vi "Write Balance.vi"(8 "error in (no error)":errorcluster, 10 "Balance":dbl, 11 "AAccount in":refnum<class "AAccount.lvclass">) -> (0 "error out":errorcluster, 3 "AAccount out":refnum<class "AAccount.lvclass">)   [LabVIEW 2020, in "AAccount.lvclass"]
uses:
  AAccount.lvclass
  AAccount.lvclass/AAccount.ctl
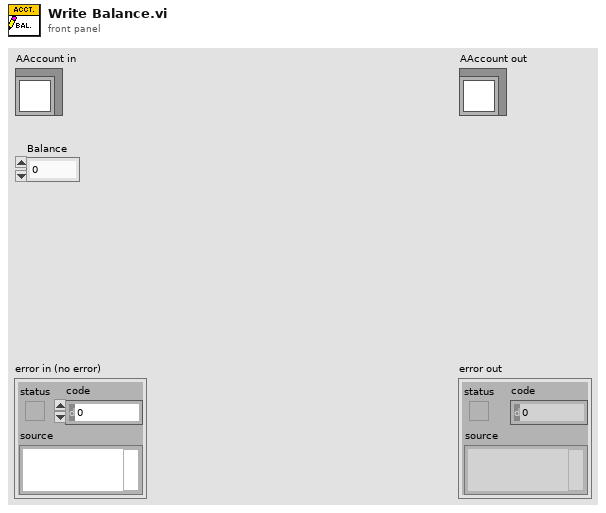
[diagram p1: front panel]
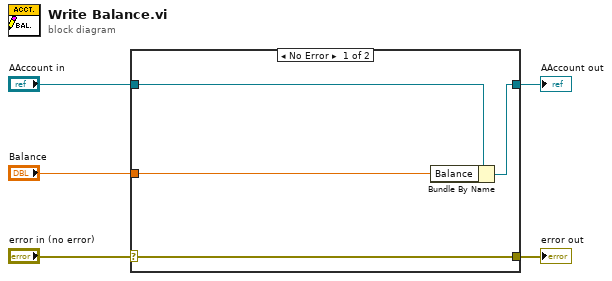
[diagram p0: block diagram]
diagram:
  n1 = case shown="No Error" "error in (no error)" {
    selector: "error in (no error)" -> [w9 w10]
    tunnel: [w9 w10] -> w4
    tunnel: [w7 w11] -> w2
    tunnel: "AAccount in" -> [w8 w11]
    tunnel: "Balance" -> [w6 _]
    frame No Error {
      n2 = Bundle By Name(cluster=w8, "Balance"=w6) -> (w7:refnum<class "AAccount.lvclass">)
    }
    frame Error {
    }
  }
  "error out" <- w4
  "AAccount out" <- w2
